vi "E8267D GetPower.vi"(0 "VISA Rsrc":refnum<visa-resource-name>="GPIB0::12::INSTR", 11 "error in (no error)":errorcluster) -> (4 "VISA Rsrc Out":refnum<visa-resource-name>="GPIB0::12::INSTR", 6 "Power (dBm)":dbl, 15 "error out":errorcluster)   [LabVIEW 2019]
doc: "Ce VI écrit les paramètres de la zone de contrôle spécifiée dans le contrôlleur"
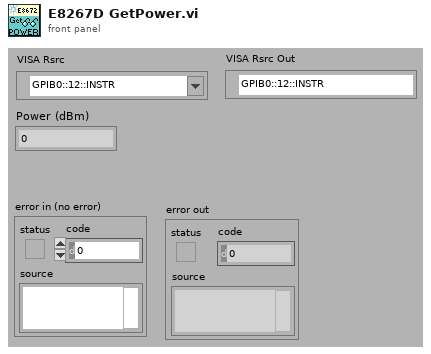
[diagram p1: front panel]
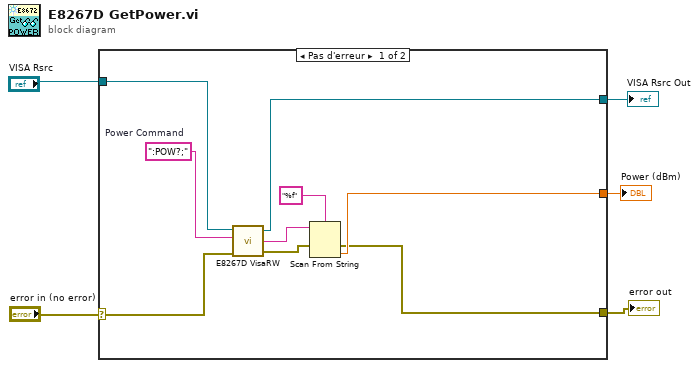
[diagram p0: block diagram]
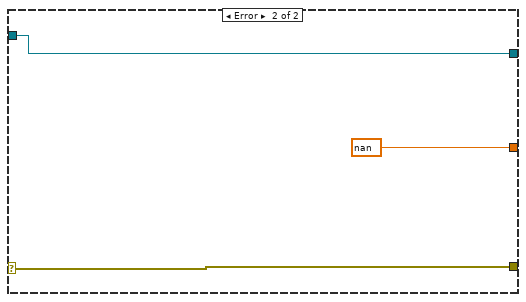
[diagram p2: hidden frame]
diagram:
  n1 = case shown="Pas d'erreur" "error in (no error)" {
    selector: "error in (no error)" -> [w14 w17]
    tunnel: "VISA Rsrc" -> [w13 w16]
    tunnel: [w7 w17] -> w4
    tunnel: [w12 w16] -> w2
    tunnel: [w8 nan] -> w1
    frame No Error {
      w11 = ":POW?;"  # Power Command
      n2 = call <userlib>:"E8267D VisaRW.vi"("error in (no error)"=w14, "ChaineCom"=w11, "VISA Rsrc"=w13) -> ("error out"=w6:errorcluster, "ChaineRep"=w10:string, "VISA Rsrc Out"=w12:refnum<visa-resource-name>)  [unwired: 4 in, 1 out]
      n3 = Scan From String(format string="%f" ("chaîne de format"), input string=w10, error in=w6) -> (error out=w7:errorcluster, output 1=w8:dbl)  [unwired: 2 in, 2 out]
    }
    frame Error {
    }
  }
  "error out" <- w4
  "Power (dBm)" <- w1
  "VISA Rsrc Out" <- w2
